vi "stop.vi"(8 "error in (no error)":errorcluster, 11 "Model in":refnum<class "Model.lvclass">) -> (0 "error out":errorcluster, 3 "Model out":refnum<class "Model.lvclass">)   [LabVIEW 2013, in "Model.lvclass"]
uses:
  Model.lvclass
  <userlib>/Common/ILC/ILC/ILC.lvclass
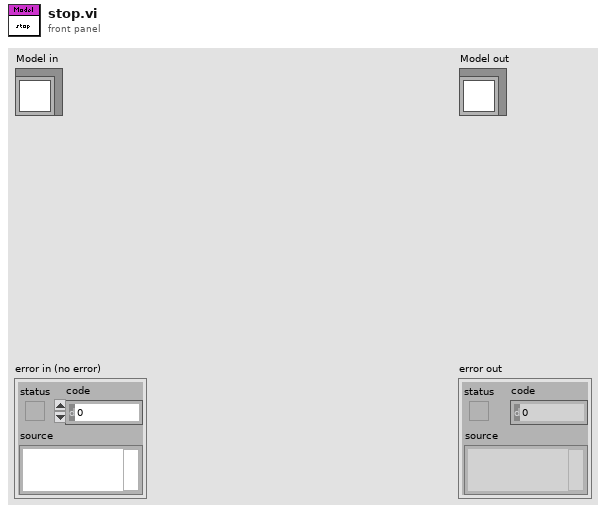
[diagram p1: front panel]
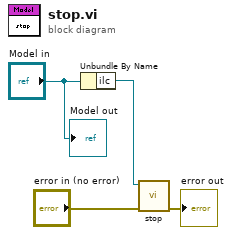
[diagram p0: block diagram]
diagram:
  n1 = Unbundle By Name("Model in") -> ("ilc"=w3:refnum<class "ILC.lvclass">)
  n2 = call <userlib>:"stop.vi"("error in (no error)"="error in (no error)", "ILC in"=w3) -> ("error out"=→"error out":errorcluster)  [unwired: 8 in, 1 out]
  "Model out" <- "Model in"
